vi "5668 Configure Triggers and Events.vi"(7 "Start Trigger":T2(ring), 8 "error in (no error)":errorcluster, 11 "Instrument Handles in":T1={"Resource Name RFSA"="RFSA", "Resource Name RFSG LO Generation"="RFSG"}) -> (0 "error out":errorcluster, 3 "Instrument Handles out":T1={"Resource Name RFSA"="RFSA", "Resource Name RFSG LO Generation"="RFSG"})   [LabVIEW 2017]
uses:
  <instrlib>/niRFSA/niRFSA.llb/niRFSA Trigger Terminals.ctl
  <instrlib>/niRFSA/niRFSA.llb/niRFSA Exported Signal Destinations.ctl
  Instrument Handles.ctl
  <instrlib>/niRFSA/niRFSA.llb/niRFSA Signal Names.ctl
  <instrlib>/niRFSA/niRFSA.llb/niRFSA Configure Software Edge Start Trigger.vi
  <instrlib>/niRFSA/niRFSA.llb/niRFSA Configure Digital Edge Start Trigger.vi
  <instrlib>/niRFSA/niRFSA.llb/niRFSA Configure Digital Edge Advance Trigger.vi
panel:
  in  "output terminal":T3="PXI_Trig1"
  in  "Start Trigger Source":T4="PXI_Trig2"
  in  "Advance Trigger Source":T4="PXI_Trig0"
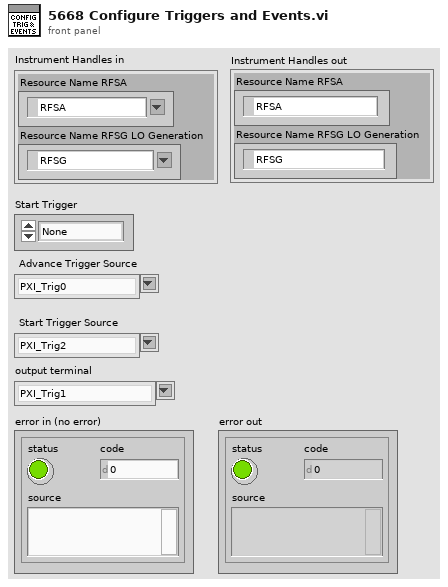
[diagram p1: front panel]
types:
  T1 = typedef "Instrument Handles.ctl" = cluster{"Resource Name RFSA":refnum<k15>, "Resource Name RFSG LO Generation":refnum<k15>}
  T2 = enum16{"None", "Software Trigger", "Hardware Trigger"}
  T3 = typedef "niRFSA Exported Signal Destinations.ctl" = string
  T4 = typedef "niRFSA Trigger Terminals.ctl" = string
  T5 = typedef "niRFSA Signal Names.ctl" = i32
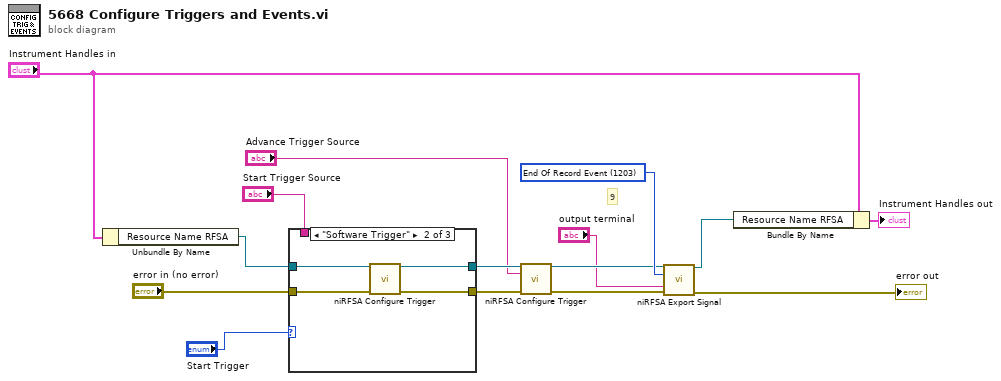
[diagram p0: block diagram]
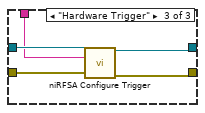
[diagram p3: hidden frame]
diagram:
  w11 = T5 1203 items=["Start Trigger"=1100, "Ref Trigger"=702, "Advance Trigger"=1102, "Ready For Start Event"=1200, "Ready For Ref Event"=1201, "Ready For Advance Event"=1202, "End Of Record Event"=1203, "Done Event"=1204, "Reference Clock"=1205, "User"=1206] ("signal")
  # "9"
  n1 = Unbundle By Name("Instrument Handles in") -> ("Resource Name RFSA"=w7:refnum<k15>)
  n2 = case shown="\"Software Trigger\"" "Start Trigger" {
    tunnel: "error in (no error)" -> [w16 w21 w26]
    tunnel: [w16 w20 w23] -> w14
    tunnel: [w17 w19 w24] -> w13
    tunnel: w7 -> [w17 w18 w25]
    tunnel: "Start Trigger Source" -> [_ _ w22]
    frame "None", Default {
    }
    frame "Software Trigger" {
      n3 = call-poly <instrlib>:"niRFSA Configure Trigger.vi"("instrument handle"=w18, "error in"=w21) -> ("instrument handle out"=w19:refnum<k15>, "error out"=w20:errorcluster)  [unwired: 12 in]
    }
    frame "Hardware Trigger" {
      n4 = call-poly <instrlib>:"niRFSA Configure Trigger.vi"("instrument handle"=w25, "source"=w22, "error in"=w26) -> ("instrument handle out"=w24:refnum<k15>, "error out"=w23:errorcluster)  [unwired: 11 in]
    }
  }
  n5 = call-poly <instrlib>:"niRFSA Configure Trigger.vi"("instrument handle"=w13, "source"="Advance Trigger Source", "error in"=w14) -> ("instrument handle out"=w10:refnum<k15>, "error out"=w9:errorcluster)  [unwired: 11 in]
  n6 = call <instrlib>:"niRFSA Export Signal.vi"("instrument handle"=w10, "signal"=w11, "output terminal"="output terminal", "error in"=w9) -> ("instrument handle out"=w6:refnum<k15>, "error out"=→"error out":errorcluster)  [unwired: 10 in]
  n7 = Bundle By Name(cluster="Instrument Handles in", "Resource Name RFSA"=w6) -> (→"Instrument Handles out":T1)
